vi "GSE 350 Send Receive.vi"(8 "error in (no error)":errorcluster, 11 "VISA Refnum in":refnum<visa-resource-name>) -> (0 "error out":errorcluster, 1 "Weight Data":string[][](array[string]), 2 "Weight (lb/kg)":dbl, 3 "VISA Refnum out":refnum<visa-resource-name>, 4 "Match Found!":bool, 5 "read buffer":string)   [LabVIEW 2016]
panel:
  out "match substring":string
  out "concatenated string":string
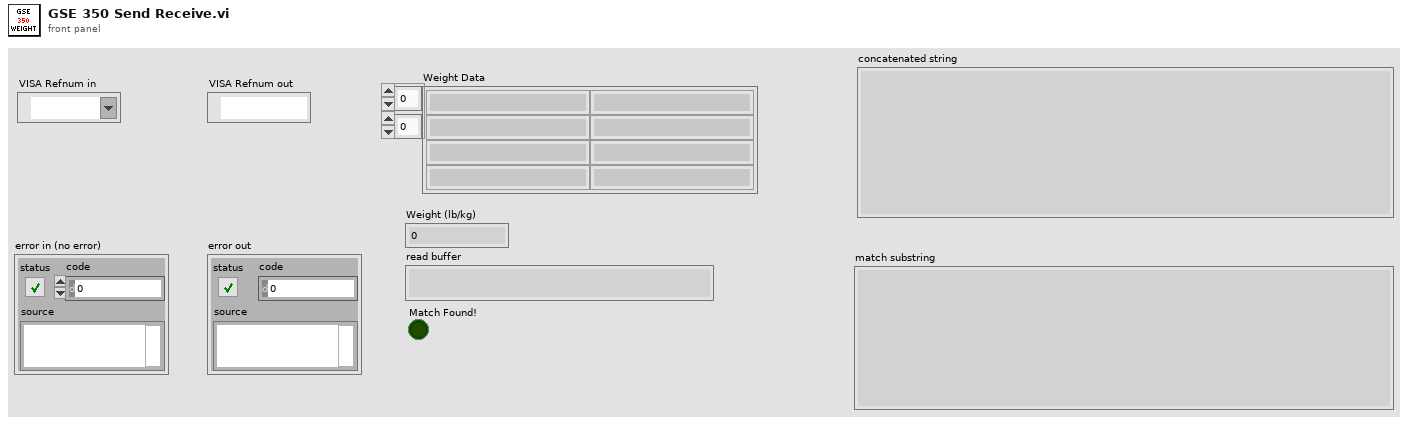
[diagram p1: front panel]
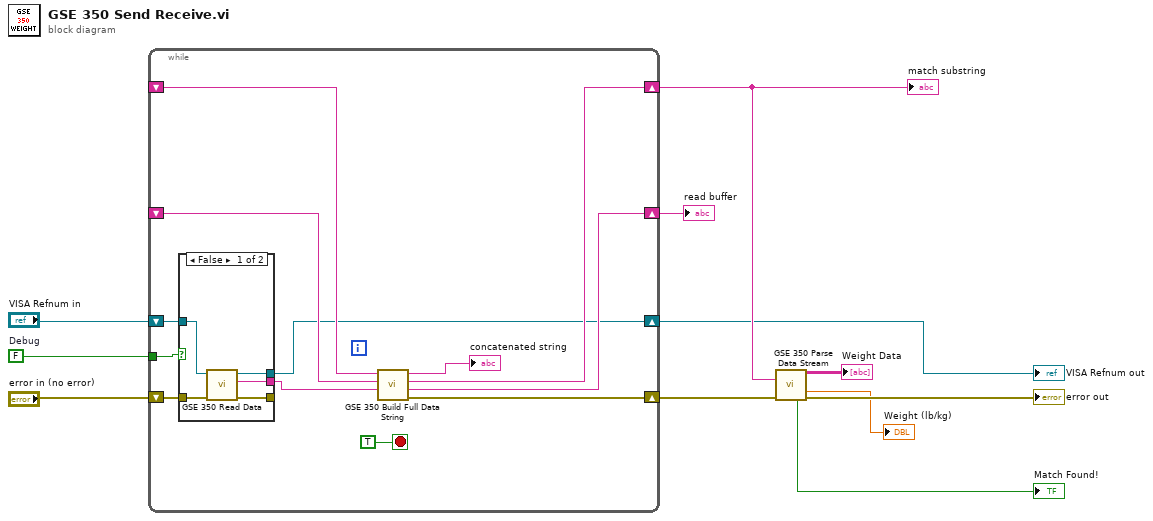
[diagram p0: block diagram]
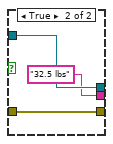
[diagram p2: hidden frame]
diagram:
  w9 = FALSE  # Debug
  n1 = while {
    tunnel: w9 -> [w21]
    shift-right: [w13] -> w7
    shift-left: "error in (no error)" -> [w23]
    shift-right: [w15] -> w4
    shift-left: "VISA Refnum in" -> [w22]
    shift-right: [w18] -> w8
    shift-left: _ -> [w19]
    shift-right: [w17] -> w6
    shift-left: _ -> [w16]
    stop <- TRUE stop-if-true
    n2 = case shown="False" w21 {
      tunnel: [w28 w31] -> w15
      tunnel: [w27 w30] -> _
      tunnel: [w24 "32.5 lbs" ("read buffer")] -> w12
      tunnel: w23 -> [w26 w30]
      tunnel: w22 -> [w25 w31]
      frame False {
        n3 = call "GSE 350 Read Data.vi"("error in (no error)"=w26, "VISA Refnum in"=w25) -> ("error out"=w27:errorcluster, "Raw Data"=w24:string, "VISA Refnum out"=w28:refnum<visa-resource-name>)  [unwired: 7 in]
      }
      frame True {
      }
    }
    n4 = call "GSE 350 Build Full Data String.vi"("Latest Data"=w12, "Previous Data"=w19, "Full Data String Input"=w16) -> ("Error Out"=w13:errorcluster, "Read Buffer (Out)"=w18:string, "Full Data String"=w17:string, "concatenated string"=→"concatenated string":string)  [unwired: 5 in]
  }
  "VISA Refnum out" <- w4
  "read buffer" <- w8
  "match substring" <- w6
  n5 = call "GSE 350 Parse Data Stream.vi"("Data Stream"=w6, "Error In"=w7) -> ("Data Array"=→"Weight Data":string[][], "Gross Weight"=→"Weight (lb/kg)":dbl, "Match Found!"=→"Match Found!":bool, "Error Out"=→"error out":errorcluster)  [unwired: 8 in, 2 out]
